vi "ResetColors.vi"(0 "AllObjs[]":refnum<vi>[](array[refnum]), 5 "Array":cluster{u32, u32}[](array[cluster])) -> ()   [LabVIEW 2014]
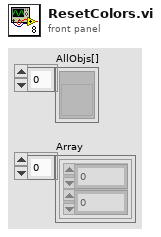
[diagram p1: front panel]
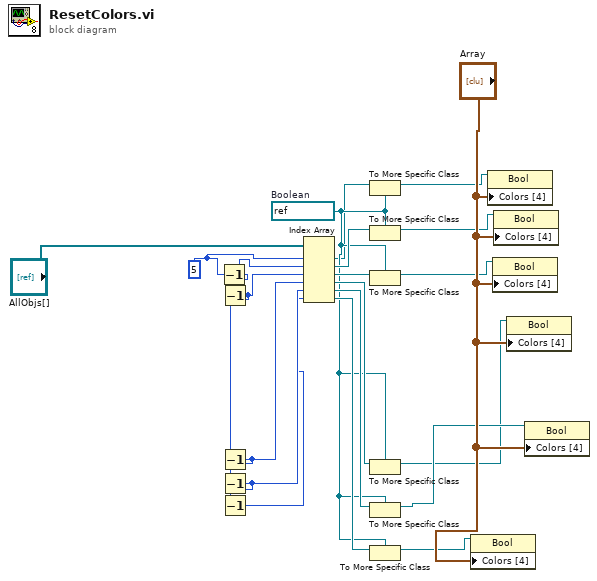
[diagram p0: block diagram]
diagram:
  w8 = refnum<vi> refnum  # Boolean
  w2 = 5
  n1 = Decrement(x=w2) -> (x-1=w4:i32)
  n2 = Decrement(x=w4) -> (x-1=w5:i32)
  n3 = Decrement(x=w5) -> (x-1=w6:i32)
  n4 = Decrement(x=w6) -> (x-1=w7:i32)
  n5 = Decrement(x=w7) -> (x-1=w3:i32)
  n6 = Index Array(array="AllObjs[]", index #1=w2, index #2=w4, index #3=w5, index #4=w6, index #5=w7, index #6=w3) -> (element #1=w1:refnum<vi>, element #2=w9:refnum<vi>, element #3=w10:refnum<vi>, element #4=w11:refnum<vi>, element #5=w12:refnum<vi>, element #6=w13:refnum<vi>)
  n7 = To More Specific Class(target class=w8, reference=w1) -> (specific class reference=w15:refnum<vi>)  [unwired: 1 in, 1 out]
  n8 = To More Specific Class(target class=w8, reference=w9) -> (specific class reference=w16:refnum<vi>)  [unwired: 1 in, 1 out]
  n9 = To More Specific Class(target class=w8, reference=w10) -> (specific class reference=w17:refnum<vi>)  [unwired: 1 in, 1 out]
  n10 = To More Specific Class(target class=w8, reference=w11) -> (specific class reference=w18:refnum<vi>)  [unwired: 1 in, 1 out]
  n11 = To More Specific Class(target class=w8, reference=w12) -> (specific class reference=w19:refnum<vi>)  [unwired: 1 in, 1 out]
  n12 = To More Specific Class(target class=w8, reference=w13) -> (specific class reference=w20:refnum<vi>)  [unwired: 1 in, 1 out]
  n13 = property class="Bool"(reference=w20, "Colors [4]"="Array") -> ()  [unwired: 1 in, 2 out]
  n14 = property class="Bool"(reference=w15, "Colors [4]"="Array") -> ()  [unwired: 1 in, 2 out]
  n15 = property class="Bool"(reference=w17, "Colors [4]"="Array") -> ()  [unwired: 1 in, 2 out]
  n16 = property class="Bool"(reference=w16, "Colors [4]"="Array") -> ()  [unwired: 1 in, 2 out]
  n17 = property class="Bool"(reference=w18, "Colors [4]"="Array") -> ()  [unwired: 1 in, 2 out]
  n18 = property class="Bool"(reference=w19, "Colors [4]"="Array") -> ()  [unwired: 1 in, 2 out]
